vi "Get Crafting Stations.vi"(8 "error in (no error)":errorcluster, 11 "Small Register Bank in":refnum<class "Small Register Bank.lvclass">) -> (0 "error out":errorcluster, 2 "Stations":T1[](array[typedef]), 3 "Small Register Bank out":refnum<class "Small Register Bank.lvclass">)   [LabVIEW 2020, in "Small Register Bank.lvclass"]
uses:
  Small Register Bank.lvclass
  Item/Craft Station.ctl
  Workstation/Workstation.lvclass
  Tinker Table/Tinker Table.lvclass
  C:/dev/IlluminatedG/lv-oopanel-gc-calc/Workstation/Workstation.lvclass
  Electronics Workbench/Electronics Workbench.lvclass
  Item/Item.lvclass
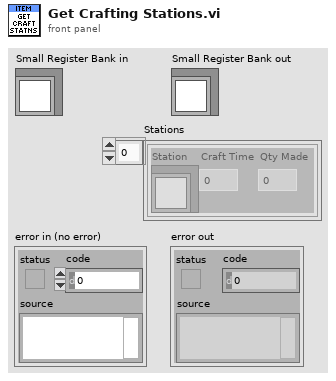
[diagram p1: front panel]
types:
  T1 = typedef "Item.lvclass/Craft Station.ctl" = cluster{"Station":refnum<class "Workstation.lvclass">, "Craft Time":dbl, "Qty Made":dbl}
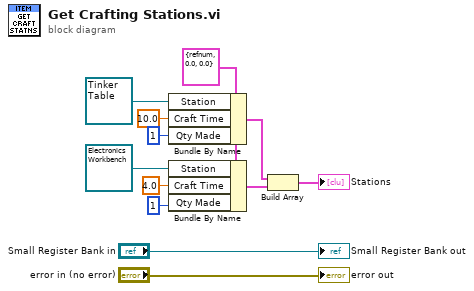
[diagram p0: block diagram]
diagram:
  w6 = T1 {"Station"=refnum, "Craft Time"=0.0, "Qty Made"=0.0} ("Craft Station")
  n1 = Bundle By Name(cluster=w6, "Station"=refnum<class "Tinker Table.lvclass"> refnum ("Tinker Table.lvclass"), "Craft Time"=10.0, "Qty Made"=1) -> (w4:T1)
  n2 = Bundle By Name(cluster=w6, "Station"=refnum<class "Electronics Workbench.lvclass"> refnum ("Electronics Workbench.lvclass"), "Craft Time"=4.0, "Qty Made"=1) -> (w5:T1)
  n3 = Build Array(w4, w5) -> (→"Stations":T1[])
  "error out" <- "error in (no error)"
  "Small Register Bank out" <- "Small Register Bank in"
